vi "Ports To System Definition.vi"(8 "error in":errorcluster, 9 "ports":T2[](array[typedef]), 10 "parameter configuration file path":path, 11 "custom device ref":T1 format="%.0x") -> (0 "error out":errorcluster, 3 "custom device ref out":T1 format="%.0x")   [LabVIEW 2020, in "ARINC 429 Scripting.lvlib"]
uses:
  ARINC 429 Scripting.lvlib
  <vilib>/NI VeriStand/Custom Device API/Custom Device Item Ref.ctl
  Shared/VS Channels Definition for All Labels on Hardware Channel.ctl
  Shared/VS Channels Definition for Label.ctl
  Shared/VS Channel Definition for Parameter.ctl
  Shared/Direction.ctl
  Shared/Parameter Definition.ctl
  Encoding and Decoding/Encoding.ctl
  Shared/Transfer Type.ctl
  <vilib>/NI VeriStand/Custom Device API/Custom Device API.lvlib
  Encoding and Decoding/Encoding and Decoding.lvlib
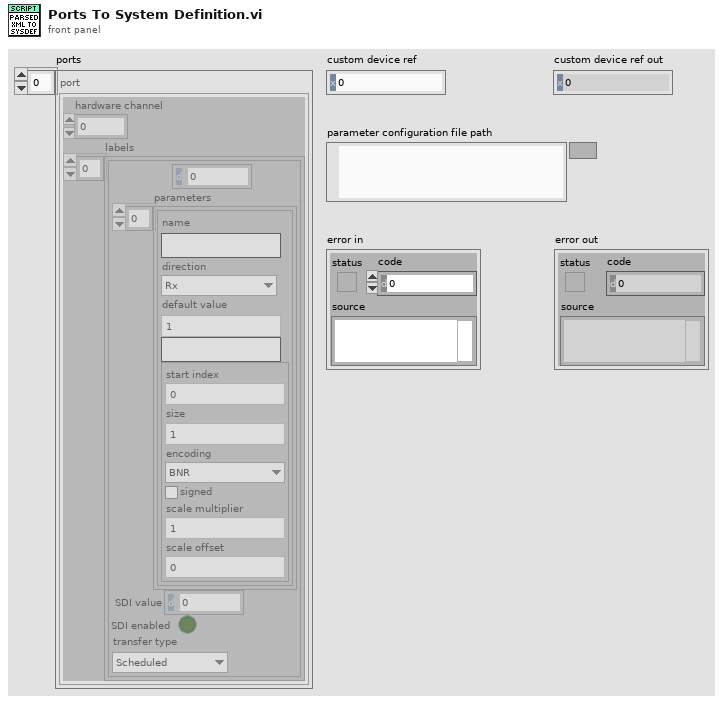
[diagram p1: front panel]
types:
  T1 = typedef "Custom Device API.lvlib/Custom Device Item Ref.ctl" = u64
  T2 = typedef "VS Channels Definition for All Labels on Hardware Channel.ctl" = cluster{"hardware channel":i32, "labels":T3[]}
  T3 = typedef "VS Channels Definition for Label.ctl" = cluster{"label (Dec)":u32, "parameters":T4[], "SDI value":u8, "SDI enabled":bool, "transfer type":T8}
  T4 = typedef "VS Channel Definition for Parameter.ctl" = cluster{"name":string, "direction":T5, "default value":dbl, "unit":string, "Parameter":T6}
  T5 = typedef "Direction.ctl" = enum16{"Rx", "Tx"}
  T6 = typedef "Parameter Definition.ctl" = cluster{"start index":i32, "size":i32, "encoding":T7, "signed":bool, "scale multiplier":dbl, "scale offset":dbl}
  T7 = typedef "Encoding and Decoding.lvlib/Encoding.ctl" = enum16{"BNR", "BCD", "Discrete"}
  T8 = typedef "Transfer Type.ctl" = enum16{"Scheduled", "Acyclic", "Block", "Strobe"}
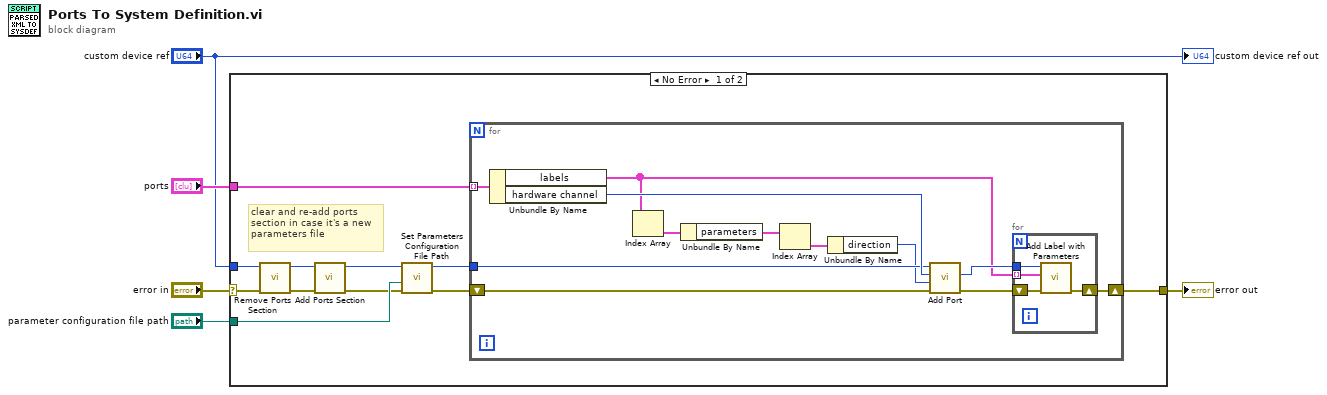
[diagram p0: block diagram]
diagram:
  n1 = case shown="No Error" "error in" {
    selector: "error in" -> [w10 w33]
    tunnel: "custom device ref" -> [w11 _]
    tunnel: [w16 w33] -> w5
    tunnel: "ports" -> [w15 _]
    tunnel: "parameter configuration file path" -> [w13 _]
    frame No Error {
      # "clear and re-add ports section in case it's a new parameters file"
      n2 = call "Remove Ports Section.vi"("error in"=w10, "custom device ref"=w11) -> ("error out"=w9:errorcluster, "custom device ref out"=w8:T1)  [unwired: 8 in]
      n3 = call "Add Ports Section.vi"("error in"=w9, "custom device ref"=w8) -> ("error out"=w6:errorcluster, "custom device ref out"=w7:T1)  [unwired: 7 in, 1 out]
      n4 = call "Set Parameters Configuration File Path.vi"("error in"=w6, "path"=w13, "custom device ref"=w7) -> ("error out"=w14:errorcluster, "custom device ref out"=w12:T1)  [unwired: 7 in]
      n5 = for {
        shift-right: [w25] -> w16
        shift-left: w14 -> [w22]
        tunnel: w12 -> [w23]
        tunnel: w15 -> [w28] mode=indexing
        n6 = Unbundle By Name(w28) -> ("labels"=w21:T3[], "hardware channel"=w24:i32)
        n7 = Index Array(array=w21) -> (element=w20:T3)  [unwired: 1 in]
        n8 = Unbundle By Name(w20) -> ("parameters"=w19:T4[])
        n9 = Index Array(array=w19) -> (element=w18:T4)  [unwired: 1 in]
        n10 = Unbundle By Name(w18) -> ("direction"=w17:T5)
        n11 = call "Add Port.vi"("error in"=w22, "direction"=w17, "port number"=w24, "custom device ref"=w23) -> ("error out"=w27:errorcluster, "port ref out"=w26:T1)  [unwired: 5 in, 1 out]
        n12 = for {
          tunnel: w26 -> [w31]
          tunnel: w21 -> [w29] mode=indexing
          shift-right: [w30] -> w25
          shift-left: w27 -> [w32]
          n13 = call "Add Label with Parameters.vi"("error in"=w32, "label"=w29, "port ref"=w31) -> ("error out"=w30:errorcluster)  [unwired: 7 in, 1 out]
        }
      }
    }
    frame Error {
    }
  }
  "error out" <- w5
  "custom device ref out" <- "custom device ref"
